vi "Seq Test Editor.vi"(6 "User Name":string="zhangxf", 8 "Sys Error":errorcluster, 9 "Part Type":string="ALL Type", 10 "Station":string="FA03", 11 "Base Path":path=path "C:/Labview Code") -> (0 "Sys Error Out":errorcluster)   [LabVIEW 2018]
uses:
  type defs/Sequence Info.ctl
  type defs/Sequence Status.ctl
  type defs/Sequence paths.ctl
  type defs/config paths for seq def.ctl
  <vilib>/Utility/file.llb/Write To Spreadsheet File (string).vi
panel:
  in  "Save":bool
  out "Sequence Name":string="F15 Audit 1 Sequence"
  in  "Exit":bool
  in  "Sequence":i32(listbox)=7
  in  "Steps":i32(listbox)
  in  "Edit Step":bool
  in  "Up":bool
  in  "Down":bool
  in  "Copy Step":bool
  in  "Delete":bool
  in  "Insert Step":bool
  # "[Page Up]"
  # "[Page Dn]"
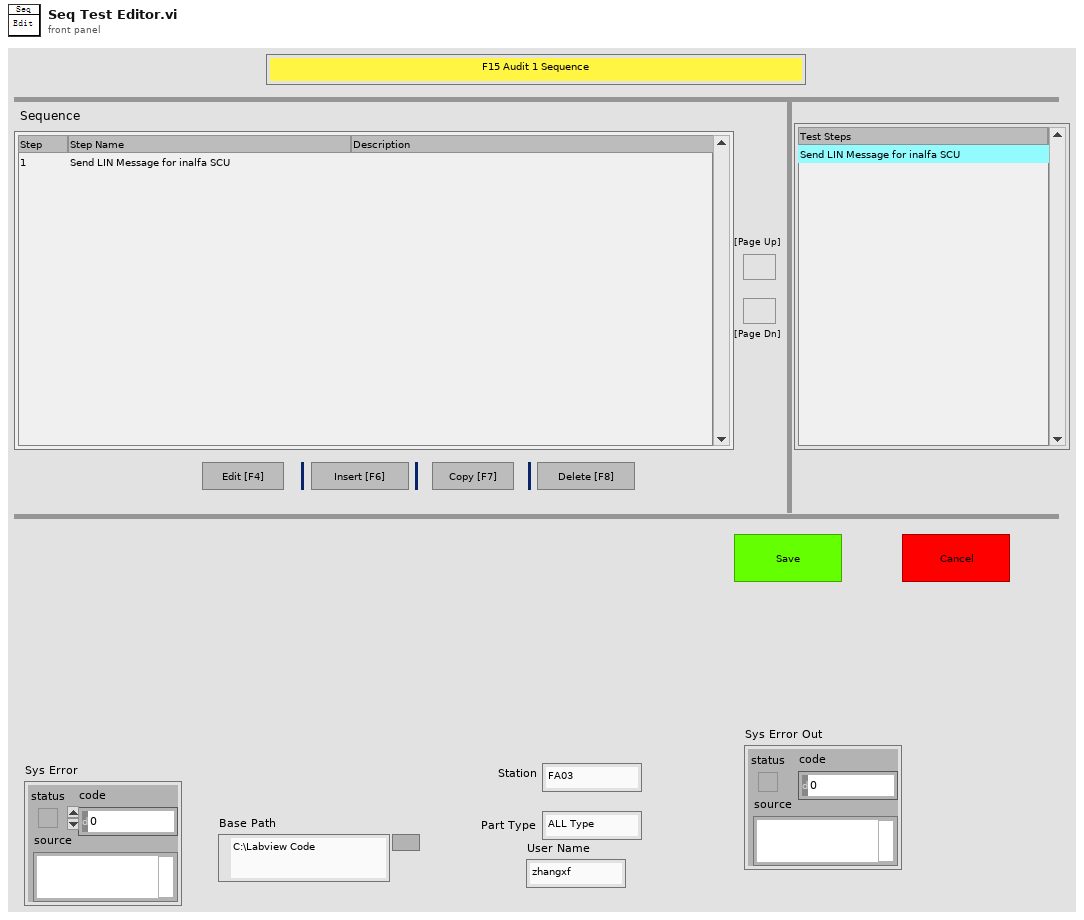
[diagram p1: front panel]
types:
  T1 = typedef "Sequence paths.ctl" = cluster{"Sequence Path":path, "Sequence Histroy Path":path, "Current Sequence Path":path, "Sequence Config Path":path, "Sequence VI's Path":path}
  T2 = typedef "Sequence Status.ctl" = enum16{"No Change", "Edited", "New Step", "Deleted", "Moved Up", "Moved Down", "Copied"}
  T3 = typedef "Sequence Info.ctl" = cluster{"Name":string, "Description":string, "data string":string}
  T4 = cluster{"Paths of Sequence":T1, "Type":string, "Sequence Name:":i32, "Sequence":refnum<vi>, "Steps":refnum<vi>, "Sequence Info":T3[], "Sequence Scroll":u32, "Basic Steps":string[], "Sequences":string[], "Sequence Text":string, "Station":string, "New Step?":bool, "Part Type":string, "User Name":string, "Sequence History":string[][], "Sequence Status":T2, "Sequence History Index":i32, "Step History Data":string[], "VI Names":string[], "Sys Error":errorcluster, "Current Sequence":string[][], "Base Path":path, "Description":string[]}
  T5 = typedef "config paths for seq def.ctl" = cluster{"Part Type":string, "base path":path, "Seq VI's path":path}
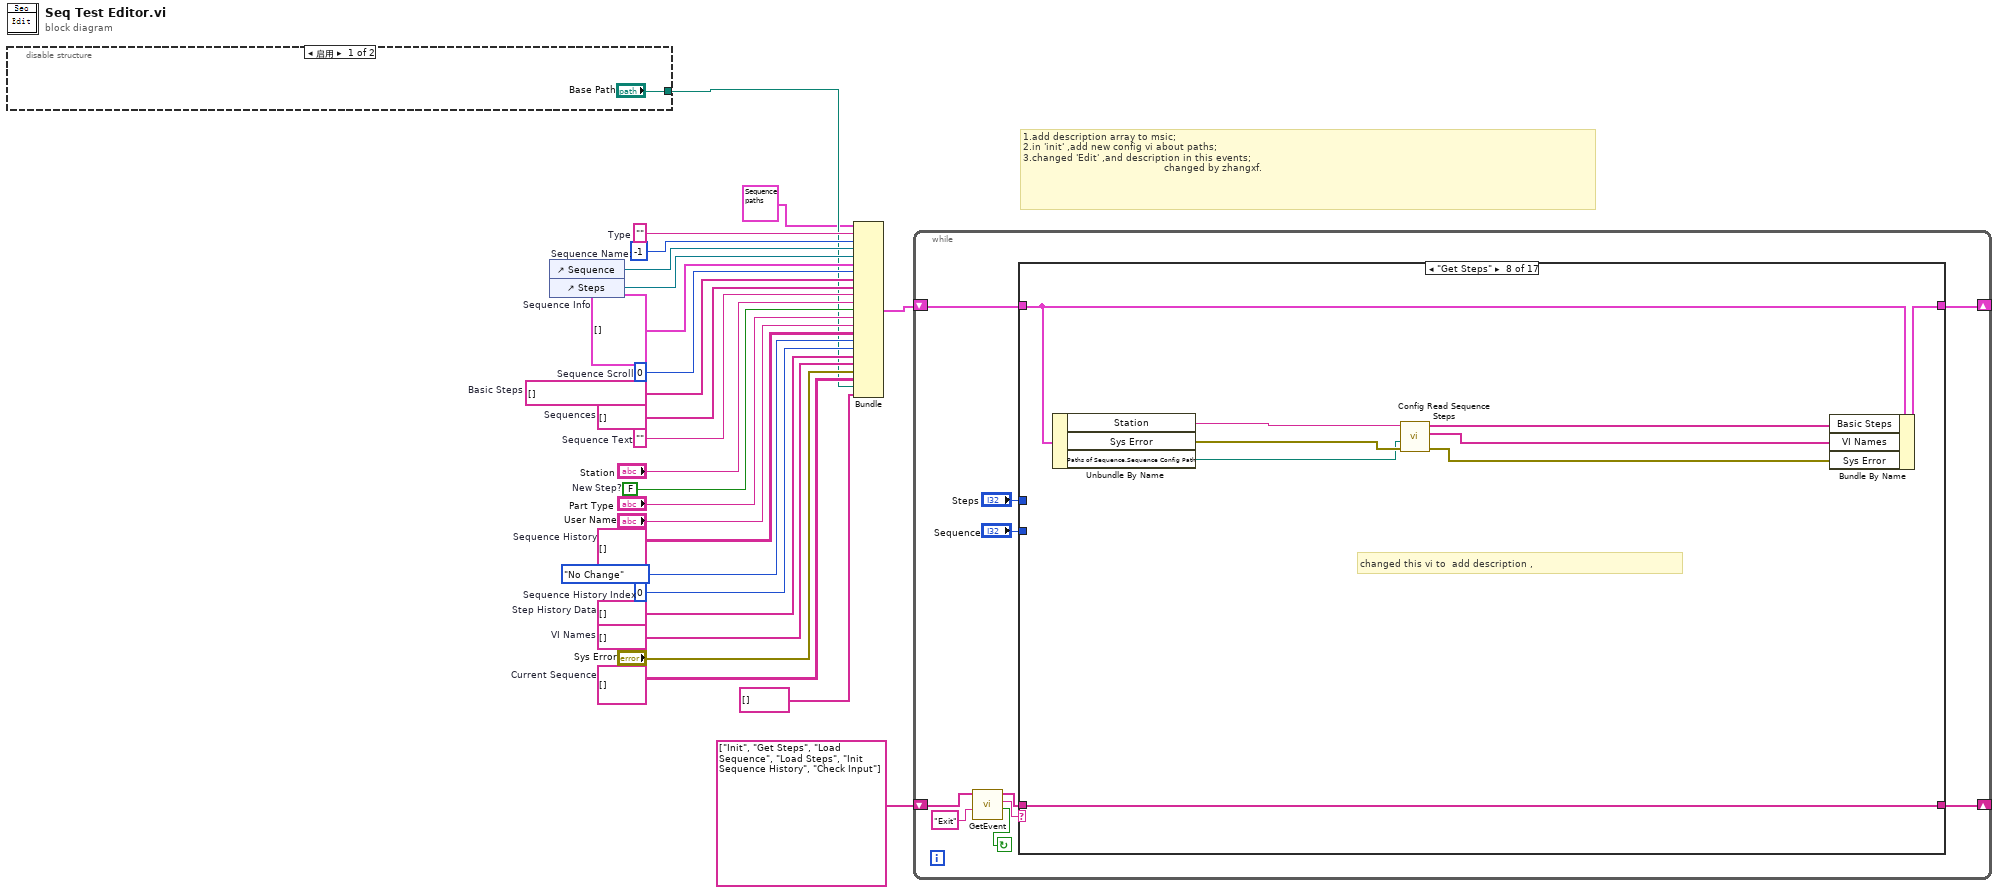
[diagram p0: block diagram]
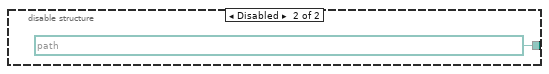
[diagram p2: hidden frame]
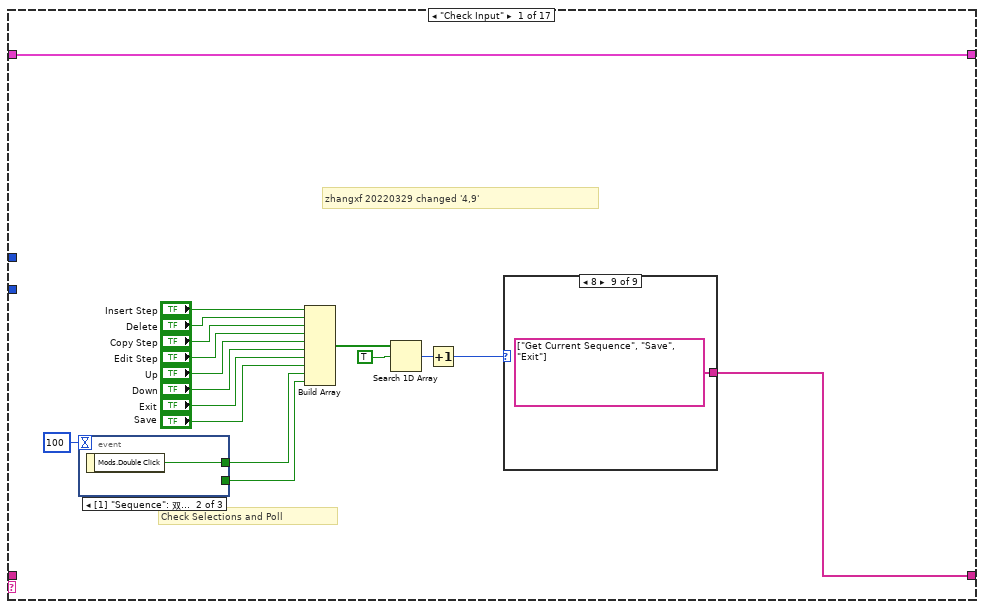
[diagram p3: hidden frame]
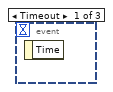
[diagram p4: hidden frame]
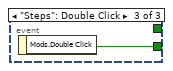
[diagram p5: hidden frame]
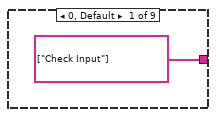
[diagram p6: hidden frame]
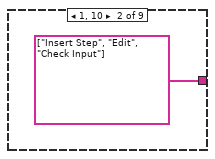
[diagram p7: hidden frame]
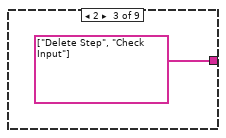
[diagram p8: hidden frame]
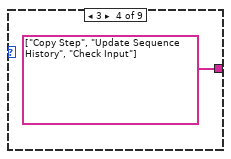
[diagram p9: hidden frame]
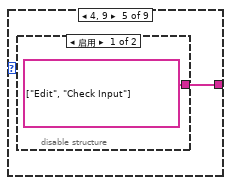
[diagram p10: hidden frame]
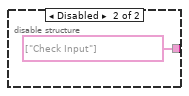
[diagram p11: hidden frame]
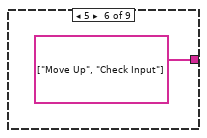
[diagram p12: hidden frame]
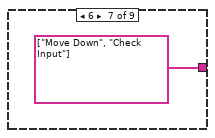
[diagram p13: hidden frame]
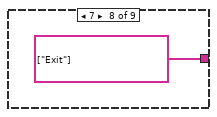
[diagram p14: hidden frame]
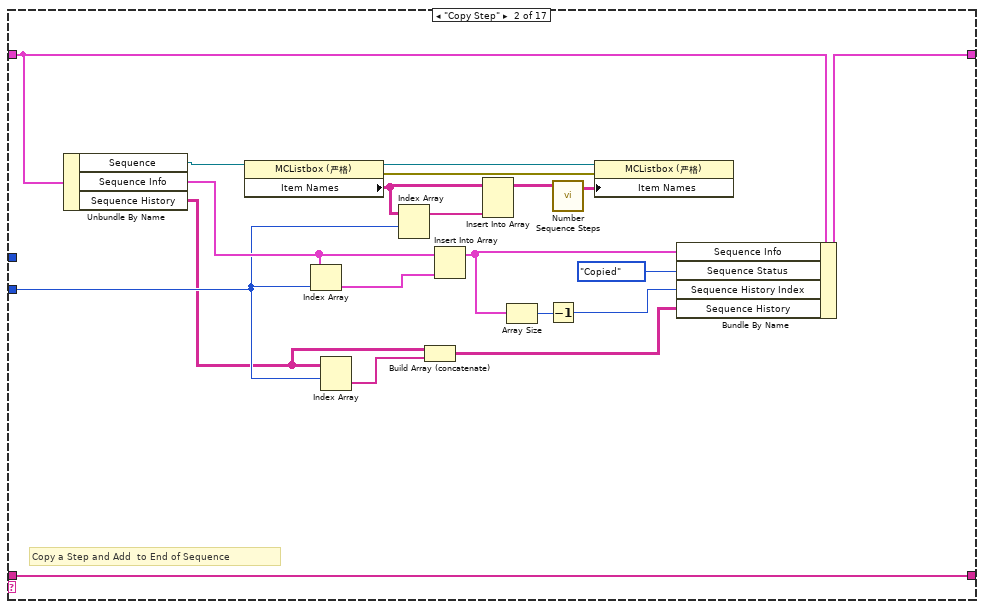
[diagram p15: hidden frame]
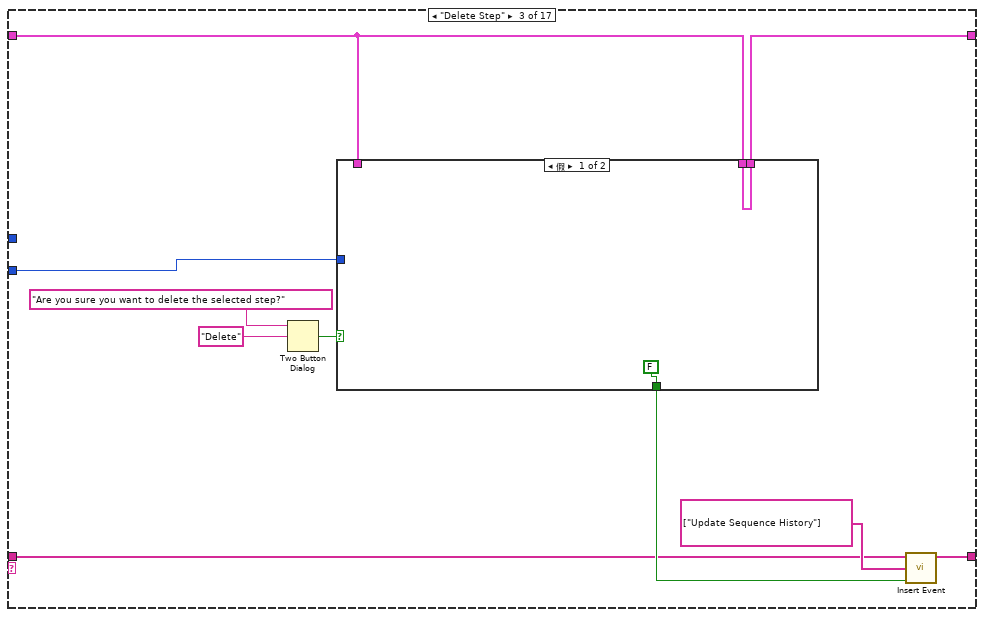
[diagram p16: hidden frame]
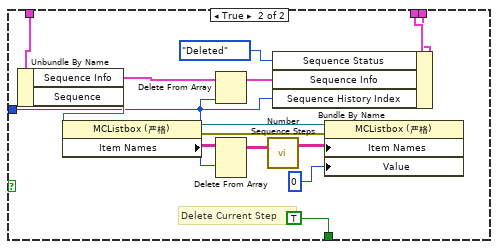
[diagram p17: hidden frame]
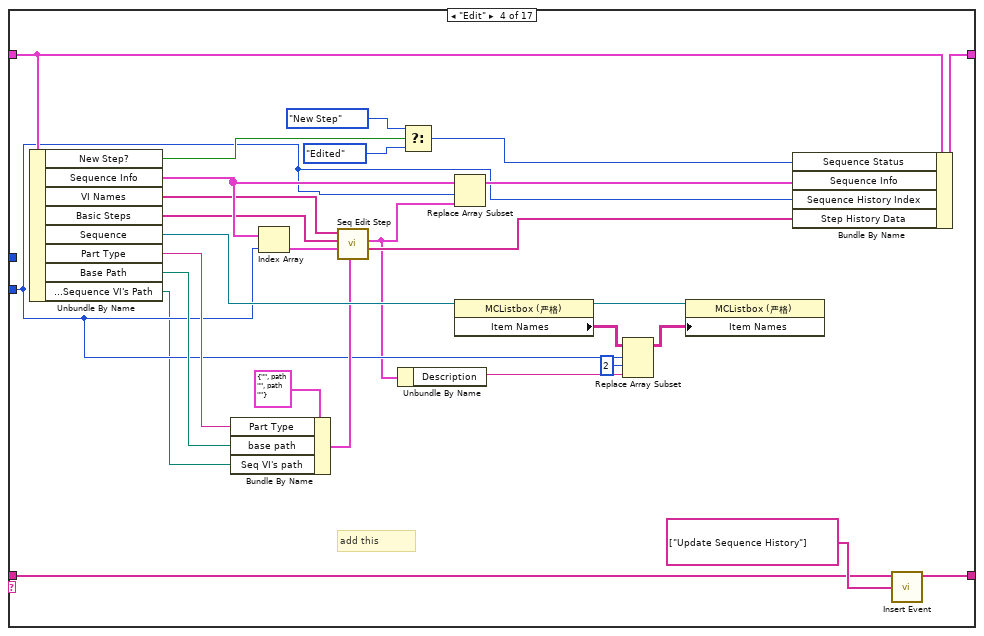
[diagram p18: hidden frame]
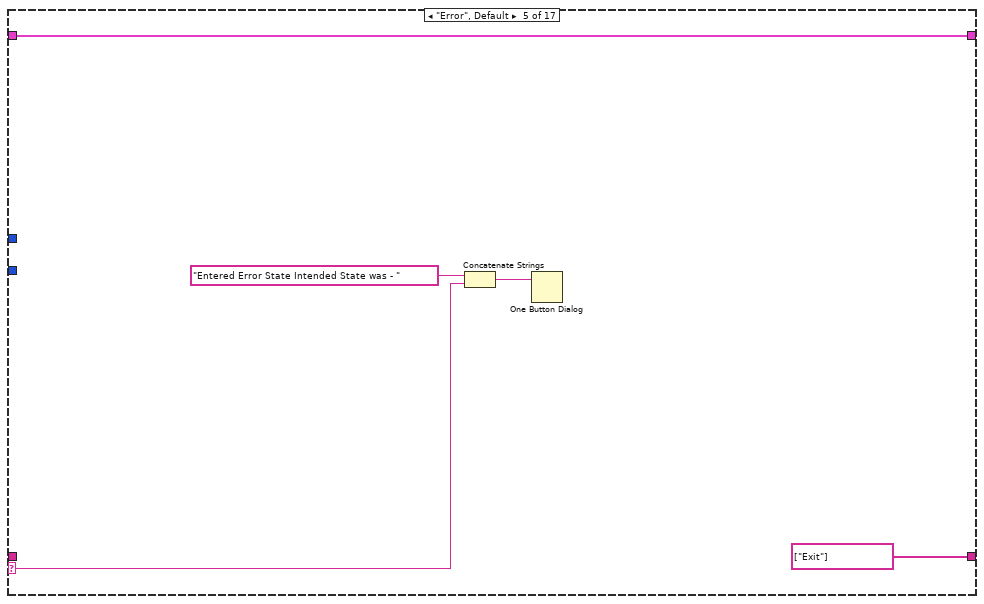
[diagram p19: hidden frame]
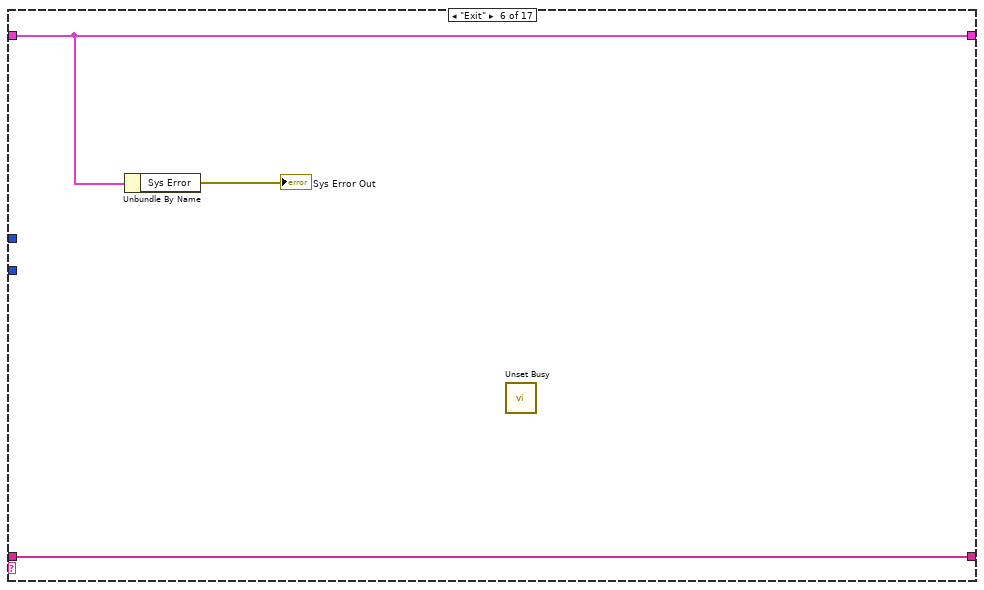
[diagram p20: hidden frame]
diagram:
  w4 = string[][] []  # Current Sequence
  w6 = string[] []  # VI Names
  w7 = string[] []  # Step History Data
  w8 = 0  # Sequence History Index
  w15 = FALSE  # New Step?
  w10 = string[][] []  # Sequence History
  w13 = T3[] []  # Sequence Info
  w17 = string[] []  # Sequences
  w19 = ""  # Sequence Text
  w20 = -1  # Sequence Name:
  w16 = string[] []  # Basic Steps
  w22 = u32 0  # Sequence Scroll
  w18 = ""  # Type
  # "1.add description array to msic;\n2.in 'init' ,add new config vi about paths;\n3.changed 'Edit' ,and description in this events;\n                                               changed by zhangxf."
  n1 = disable-structure shown="启用" {
    disable-tunnel: ["Base Path" path "D:/工作盘/116所/RD246/NI/RD246_MES/Mobitech_MES/System/Part Configuration" ("Base Path")] -> w3
    frame Enabled {
    }
    frame Disabled {
    }
  }
  n2 = control-ref of="Sequence"() -> (w23:refnum<vi>)
  n3 = control-ref of="Steps"() -> (w21:refnum<vi>)
  n4 = Bundle("Paths of Sequence"=T1 {"Sequence Path"=path "", "Sequence Histroy Path"=path "", "Current Sequence Path"=path "", "Sequence Config Path"=path "", "Sequence VI's Path"=path ""}, "Type"=w18, "Sequence Name:"=w20, "Sequence"=w23, "Steps"=w21, "Sequence Info"=w13, "Sequence Scroll"=w22, "Basic Steps"=w16, "Sequences"=w17, "Sequence Text"=w19, "Station"="Station", "New Step?"=w15, "Part Type"="Part Type", "User Name"="User Name", "Sequence History"=w10, "Sequence Status"=Sequence_Status."No Change", "Sequence History Index"=w8, "Step History Data"=w7, "VI Names"=w6, "Sys Error"="Sys Error", "Current Sequence"=w4, "Base Path"=w3, "Description"=string[] []) -> (w24:T4)  [unwired: 1 in]
  n5 = while {
    shift-right: [w37] -> _
    shift-left: string[] ["Init", "Get Steps", "Load Sequence", "Load Steps", "Init Sequence History", "Check Input"] -> [w32]
    shift-right: [w35] -> _
    shift-left: w24 -> [w36]
    stop <- w30 continue-if-true
    n6 = call "GetEvent.vi"("标志事件"="Exit" ("Exit Event"), "事件组"=w32) -> ("？"=w30:bool, "下一事件"=w28:string, "下一事件组"=w29:string[])  [unwired: 3 in, 2 out]
    n7 = case shown="\"Get Steps\"" w28 {
      selector: w28 -> [_ _ _ _ w144 _ _ _ _ _ _ _ _ _ _ _ _]
      tunnel: w29 -> [_ w80 w88 w129 _ w150 w162 w183 w193 w208 w224 w256 w264 w266 w302 w335 w350]
      tunnel: [w47 w80 w89 w130 string[] ["Exit"] ("event queue out") w150 w162 w183 w193 w208 w224 w256 w264 w267 w301 w335 w350] -> w37
      tunnel: w36 -> [w40 w82 w94 w142 w147 w149 w158 w182 w185 w198 w234 w254 w259 w277 w304 w340 w347]
      tunnel: [w40 w81 w93 w141 w147 w149 w157 w181 w186 w197 w233 w258 w259 w279 w306 w340 w349] -> w35
      tunnel: "Steps" -> [_ _ _ _ _ _ _ _ _ _ w220 _ _ _ _ _ _]
      tunnel: "Sequence" -> [_ w72 w92 w119 _ _ _ _ _ _ w223 _ _ w271 w305 _ _]
      frame "Check Input" {
        # "zhangxf 20220329 changed '4,9'"
        # "Check Selections and Poll"
        n8 = event shown="[1] \"Sequence\": 双击" {
          selector: _ -> [_ _ _]
          dyn-events: _ -> [_ _ _]
          timeout: 100 -> [_ _ _]
          tunnel: [_ w55 _] -> w44
          tunnel: [_ _ w56] -> w43
          event Timeout {
            n9 = event-data() -> ()  [unwired: 1 in, 1 out]
          }
          event "Sequence": Double Click {
            n10 = event-data() -> ("Mods.Double Click"=w55:bool)  [unwired: 1 in]
          }
          event "Steps": Double Click {
            n11 = event-data() -> ("Mods.Double Click"=w56:bool)  [unwired: 1 in]
          }
        }
        n12 = Build Array("Insert Step", "Delete", "Copy Step", "Edit Step", "Up", "Down", "Exit", "Save", w44, w43) -> (w50:bool[])
        n13 = Search 1D Array(1D array=w50, element=TRUE) -> (index of element=w49:i32)  [unwired: 1 in]
        n14 = Increment(x=w49) -> (x+1=w38:i32)
        n15 = case shown="8" w38 {
          tunnel: [string[] ["Check Input"] string[] ["Insert Step", "Edit", "Check Input"] string[] ["Delete Step", "Check Input"] string[] ["Copy Step", "Update Sequence History", "Check Input"] w61 string[] ["Move Up", "Check Input"] string[] ["Move Down", "Check Input"] string[] ["Exit"] string[] ["Get Current Sequence", "Save", "Exit"]] -> w47
          frame 0, Default {
          }
          frame 1, 10 {
          }
          frame 2 {
          }
          frame 3 {
          }
          frame 4, 9 {
            n16 = disable-structure shown="启用" {
              disable-tunnel: [string[] ["Edit", "Check Input"] string[] ["Check Input"]] -> w61
              frame Enabled {
              }
              frame Disabled {
              }
            }
          }
          frame 5 {
          }
          frame 6 {
          }
          frame 7 {
          }
          frame 8 {
          }
        }
      }
      frame "Copy Step" {
        # "Copy a Step and Add  to End of Sequence"
        n17 = Unbundle By Name(w82) -> ("Sequence"=w87:refnum<vi>, "Sequence Info"=w77:T3[], "Sequence History"=w71:string[][])
        n18 = property class="MCListbox (严格)"(reference=w87) -> (reference out=w84:refnum<vi>, error out=w83:errorcluster, "Item Names"=w79:string[][])  [unwired: 1 in]
        n19 = Index Array(array=w77, index=w72) -> (element=w76:T3)
        n20 = Index Array(array=w71, index (row)=w72) -> (element=w70:string[])  [unwired: 1 in]
        n21 = Index Array(array=w79, index (row)=w72) -> (element=w78:string[])  [unwired: 1 in]
        n22 = Build Array (concatenate)(w71, w70) -> (w69:string[][])
        n23 = Insert Into Array(array=w77, new element=w76) -> (w68:T3[])  [unwired: 1 in]
        n24 = Insert Into Array(array=w79, new element=w78) -> (w86:string[][])  [unwired: 2 in]
        n25 = Array Size(array=w68) -> (size(s)=w74:i32)
        n26 = Decrement(x=w74) -> (x-1=w73:i32)
        n27 = call "Number Sequence Steps.vi"("Sequence Names"=w86) -> ("ItemNames Out"=w85:string[][])  [unwired: 1 out]
        n28 = property class="MCListbox (严格)"(reference=w84, error in=w83, "Item Names"=w85) -> ()  [unwired: 2 out]
        n29 = Bundle By Name(cluster=w82, "Sequence Info"=w68, "Sequence Status"=Sequence_Status."Copied", "Sequence History Index"=w73, "Sequence History"=w69) -> (w81:T4)
      }
      frame "Delete Step" {
        n30 = Two Button Dialog(message="Are you sure you want to delete the selected step?", 2:"Delete" ("T button name (\"OK\")")) -> (T button?=w95:bool)  [unwired: 1 in]
        n31 = case shown="假" w95 {
          tunnel: w94 -> [_ w114]
          tunnel: w94 -> [w99 w112]
          tunnel: [w99 w111] -> w93
          tunnel: w92 -> [_ w101]
          tunnel: [FALSE TRUE] -> w90
          frame False {
          }
          frame True {
            # "Delete Current Step"
            n32 = Unbundle By Name(w114) -> ("Sequence Info"=w110:T3[], "Sequence"=w113:refnum<vi>)
            n33 = property class="MCListbox (严格)"(reference=w113) -> (reference out=w107:refnum<vi>, error out=w106:errorcluster, "Item Names"=w108:string[][])  [unwired: 1 in]
            n34 = Delete From Array(array=w110, index=w101) -> (array with subset deleted=w109:T3[])  [unwired: 1 in, 1 out]
            n35 = Delete From Array(array=w108, index (row)=w101) -> (array with subset deleted=w105:string[][])  [unwired: 2 in, 1 out]
            n36 = call "Number Sequence Steps.vi"("Sequence Names"=w105) -> ("ItemNames Out"=w104:string[][])  [unwired: 1 out]
            n37 = Bundle By Name(cluster=w112, "Sequence Status"=Sequence_Status."Deleted", "Sequence Info"=w109, "Sequence History Index"=w101) -> (w111:T4)
            n38 = property class="MCListbox (严格)"(reference=w107, error in=w106, "Item Names"=w104, "Value"=0) -> ()  [unwired: 2 out]
          }
        }
        n39 = call "Insert Event.vi"("Event queue in"=w88, "Insert all? (T)"=w90, "Events to Insert"=string[] ["Update Sequence History"]) -> ("Event queue out"=w89:string[])  [unwired: 7 in]
      }
      frame "Edit" {
        # "add this"
        n40 = Unbundle By Name(w142) -> ("New Step?"=w136:bool, "Sequence Info"=w139:T3[], "VI Names"=w128:string[], "Basic Steps"=w126:string[], "Sequence"=w127:refnum<vi>, "Part Type"=w124:string, "Base Path"=w123:path, "Paths of Sequence.Sequence VI's Path"=w115:path)
        n41 = Bundle By Name(cluster=T5 {"Part Type"="", "base path"=path "", "Seq VI's path"=path ""} ("config paths"), "Part Type"=w124, "base path"=w123, "Seq VI's path"=w115) -> (w122:T5)
        n42 = Index Array(array=w139, index=w119) -> (element=w137:T3)
        n43 = call "Seq Edit Step.vi"("config paths"=w122, "Segment Info In"=w137, "Basic Steps"=w126, "VI Names"=w128) -> ("Step Hisitory"=w132:string[], "Segment Info Out"=w118:T3)  [unwired: 4 in, 2 out]
        n44 = Unbundle By Name(w118) -> ("Description"=w117:string)
        n45 = Select(t=Sequence_Status."New Step" ("Sequence Status"), s=w136, f=Sequence_Status."Edited" ("Sequence Status")) -> (s? t:f=w133:T2)
        n46 = Replace Array Subset(array=w139, new element=w118, index=w119) -> (w140:T3[])
        n47 = property class="MCListbox (严格)"(reference=w127) -> (reference out=w138:refnum<vi>, "Item Names"=w121:string[][])  [unwired: 1 in, 1 out]
        n48 = Replace Array Subset(array=w121, new element=w117, index (row)=w119, index (col)=2 ("禁用的索引 (列)")) -> (w120:string[][])
        n49 = property class="MCListbox (严格)"(reference=w138, "Item Names"=w120) -> ()  [unwired: 1 in, 2 out]
        n50 = Bundle By Name(cluster=w142, "Sequence Status"=w133, "Sequence Info"=w140, "Sequence History Index"=w119, "Step History Data"=w132) -> (w141:T4)
        n51 = call "Insert Event.vi"("Event queue in"=w129, "Events to Insert"=string[] ["Update Sequence History"]) -> ("Event queue out"=w130:string[])  [unwired: 8 in]
      }
      frame "Error", Default {
        n52 = Concatenate Strings("Entered Error State Intended State was - " ("string"), w144) -> (w143:string)
        n53 = One Button Dialog(message=w143) -> ()  [unwired: 1 in, 1 out]
      }
      frame "Exit" {
        n54 = Unbundle By Name(w149) -> ("Sys Error"=→"Sys Error Out":errorcluster)
        n55 = call <vilib>:"Unset Busy.vi"() -> ()  [unwired: 11 in, 1 out]
      }
      frame "Get Current Sequence" {
        n56 = Unbundle By Name(w158) -> ("VI Names"=w159:string[], "Basic Steps"=w160:string[], "Sequence Info"=w161:T3[], "Part Type"=w154:string, "Base Path"=w153:path, "Paths of Sequence.Sequence VI's Path"=w151:path)
        n57 = Bundle By Name(cluster=T5 {"Part Type"="", "base path"=path "", "Seq VI's path"=path ""} ("config paths"), "Part Type"=w154, "base path"=w153, "Seq VI's path"=w151) -> (w152:T5)
        n58 = for {
          tunnel: w161 -> [w174] mode=indexing
          tunnel: w160 -> [w173]
          tunnel: w159 -> [w172]
          tunnel: [w167] -> w156 mode=indexing
          tunnel: w152 -> [w163]
          n59 = call "Seq Get Current Sequence.vi"("config paths"=w163, "Segment Info In"=w174, "Basic Steps"=w173, "VI Names"=w172) -> ("Step Hisitory"=w171:string[])  [unwired: 6 in, 1 out]
          n60 = Index Array(array=w171, index #1=0 ("index"), index #2=3 ("index"), index #3=1 ("index")) -> (element #1=w170:string, element #2=w169:string, element #3=w168:string)
          n61 = Build Array(w170, w169, w168) -> (w167:string[])
        }
        n62 = call <vilib>:"Set Busy.vi"() -> ()  [unwired: 10 in, 2 out]
        n63 = Bundle By Name(cluster=w158, "Current Sequence"=w156) -> (w157:T4)
      }
      frame "Get Steps" {
        # "changed this vi to  add description ,"
        n64 = Unbundle By Name(w182) -> ("Station"=w180:string, "Sys Error"=w177:errorcluster, "Paths of Sequence.Sequence Config Path"=w175:path)
        n65 = call "Config Read Sequence Steps.vi"("Error In"=w177, "Base Path"=w175, "Station Name"=w180) -> ("Error Out"=w176:errorcluster, "VI Names"=w178:string[], "Sequence Steps"=w179:string[])  [unwired: 6 in]
        n66 = Bundle By Name(cluster=w182, "Basic Steps"=w179, "VI Names"=w178, "Sys Error"=w176) -> (w181:T4)
      }
      frame "Init" {
        w190 = string[][] [] ("Item Names")
        w189 = u32 9567230
        w188 = 0 ("Value")
        # "add this vi to config paths"
        n67 = Unbundle By Name(w185) -> ("Sequence"=w192:refnum<vi>, "Steps"=w191:refnum<vi>)
        n68 = call "Creat file for Seq path.vi"("ini in"=w185) -> ("Paths of Sequence"=w184:T1)  [unwired: 10 in]
        n69 = property class="MCListbox (严格)"(reference=w192, "Item Names"=w190, "Value"=w188, "Selection Color"=w189) -> ()  [unwired: 1 in, 2 out]
        n70 = property class="MCListbox (严格)"(reference=w191, "Item Names"=w190, "Value"=w188, "Selection Color"=w189, "Disabled Items"=i32[] []) -> ()  [unwired: 1 in, 2 out]
        n71 = Bundle By Name(cluster=w185, "Paths of Sequence"=w184) -> (w186:T4)
      }
      frame "Init Sequence History" {
        n72 = Unbundle By Name(w198) -> ("User Name"=w202:string, "Part Type"=w204:string, "Station"=w206:string, "Sequence Info"=w207:T3[], "Sequence Status"=w195:T2)
        n73 = Get Date/Time String() -> (date string=w200:string, time string=w201:string)  [unwired: 3 in]
        n74 = Format Into String(w204) -> (resulting string=w203:string)  [unwired: 3 in, 1 out]
        n75 = Format Into String(w206) -> (resulting string=w205:string)  [unwired: 3 in, 1 out]
        n76 = Format Into String(w195) -> (resulting string=w199:string)  [unwired: 3 in, 1 out]
        n77 = for {
          tunnel: w207 -> [w218] mode=indexing
          tunnel: w205 -> [w213]
          tunnel: w203 -> [w214]
          tunnel: w202 -> [w215]
          tunnel: w201 -> [w216]
          tunnel: w200 -> [w217]
          tunnel: [w211] -> w196 mode=indexing
          tunnel: w199 -> [w210]
          tunnel: "NA" -> [w209]
          n78 = Unbundle By Name(w218) -> ("Name"=w212:string)
          n79 = Build Array(w215, w217, w216, w214, w213, w212, w210, w209, w209) -> (w211:string[])
        }
        n80 = Bundle By Name(cluster=w198, "Sequence History"=w196) -> (w197:T4)
      }
      frame "Insert Step" {
        # "zhangxf 20220328 changed: This change causes the new \nstep to be inserted downward"
        # "zhangxf 20220328 changed: add description in items"
        n81 = Unbundle By Name(w234) -> ("Sequence"=w242:refnum<vi>, "Steps"=w245:refnum<vi>, "Sequence Info"=w229:T3[], "Description"=w221:string[])
        n82 = property class="MCListbox (严格)"(reference=w245) -> (error out=w241:errorcluster, "Item Names"=w244:string[][])  [unwired: 1 in, 1 out]
        n83 = Index Array(array=w221, index=w220) -> (element=w219:string)
        n84 = case shown="..-1" w223 {
          selector: w223 -> [w247 _]
          tunnel: [w246 0 ("Sequence")] -> w222
          frame 0.. {
            n85 = Increment(x=w247) -> (x+1=w246:i32)
          }
          frame ..-1 {
          }
        }
        n86 = Index Array(array=w244, index (row)=w220, index (col)=0 ("disabled index (col)")) -> (element=w228:string)
        n87 = property class="MCListbox (严格)"(reference=w242, error in=w241) -> (reference out=w236:refnum<vi>, error out=w235:errorcluster, "Item Names"=w239:string[][])
        n88 = Bundle By Name(cluster=T3 {"Name"="", "Description"="", "data string"=""} ("Segment Data"), "Name"=w228, "Description"=w219) -> (w231:T3)
        n89 = Build Array("1" ("element"), w228, "") -> (w238:string[])
        n90 = Insert Into Array(array=w239, index (row)=w222, new element=w238) -> (w240:string[][])  [unwired: 1 in]
        n91 = Insert Into Array(array=w229, index=w222, new element=w231) -> (w230:T3[])
        n92 = call "Number Sequence Steps.vi"("Sequence Names"=w240) -> ("ItemNames Out"=w237:string[][])  [unwired: 1 out]
        n93 = property class="MCListbox (严格)"(reference=w236, error in=w235, "Item Names"=w237, "Value"=w222) -> ()  [unwired: 2 out]
        n94 = Bundle By Name(cluster=w234, "Sequence Info"=w230, "New Step?"=TRUE) -> (w233:T4)
      }
      frame "Load Sequence" {
        # "Load Sequence"
        n95 = Unbundle By Name(w254) -> ("Sequence"=w257:refnum<vi>, "Part Type"=w250:string, "Station"=w251:string, "Paths of Sequence.Sequence Path"=w249:path)
        n96 = call "Config Load Sequence.vi"("Base Path"=w249, "Station"=w251, "Part Type"=w250) -> ("Sequence Name"=→"Sequence Name":string, "Item Names"=w255:string[][], "Seqence Info"=w253:T3[])  [unwired: 5 in, 1 out]
        n97 = property class="MCListbox (严格)"(reference=w257, "Item Names"=w255) -> ()  [unwired: 1 in, 2 out]
        n98 = Bundle By Name(cluster=w254, "Sequence Info"=w253) -> (w258:T4)
      }
      frame "Load Steps" {
        n99 = Unbundle By Name(w259) -> ("Steps"=w263:refnum<vi>, "Basic Steps"=w262:string[])
        n100 = Build Array(w262) -> (w261:string[][])
        n101 = Transpose 2D Array(2D array=w261) -> (transposed array=w260:string[][])
        n102 = property class="MCListbox (严格)"(reference=w263, "Item Names"=w260) -> ()  [unwired: 1 in, 2 out]
      }
      frame "Move Down" {
        # "Move the step Down one in the sequence"
        n103 = Unbundle By Name(w277) -> ("Sequence Info"=w276:T3[], "Sequence"=w275:refnum<vi>)
        n104 = property class="MCListbox (严格)"(reference=w275) -> (reference out=w280:refnum<vi>, error out=w278:errorcluster, "Item Names"=w274:string[][])  [unwired: 1 in]
        n105 = Array Size(array=w274) -> (size(s)=w273:i32[])
        n106 = Index Array(array=w273) -> (element=w272:i32)  [unwired: 1 in]
        n107 = Decrement(x=w272) -> (x-1=w269:i32)
        n108 = Greater?(x=w269, y=w271) -> (0:w270:bool)
        n109 = case shown="真" w270 {
          tunnel: w280 -> [_ w299]
          tunnel: [w282 w298] -> w279
          tunnel: w278 -> [_ w297]
          tunnel: w277 -> [w282 w296]
          tunnel: w276 -> [_ w295]
          tunnel: w274 -> [_ w291]
          tunnel: w271 -> [_ w284]
          tunnel: [FALSE TRUE] -> w265
          frame False {
            # "At Bottom"
          }
          frame True {
            # "Move Down"
            n110 = Delete From Array(array=w295, index=w284) -> (deleted portion=w293:T3, array with subset deleted=w294:T3[])  [unwired: 1 in]
            n111 = Delete From Array(array=w291, index (row)=w284) -> (deleted portion=w289:string[], array with subset deleted=w290:string[][])  [unwired: 2 in]
            n112 = Increment(x=w284) -> (x+1=w288:i32)
            n113 = Insert Into Array(array=w294, index=w288, new element=w293) -> (w292:T3[])
            n114 = Insert Into Array(array=w290, index (row)=w288, new element=w289) -> (w287:string[][])  [unwired: 1 in]
            n115 = Bundle By Name(cluster=w296, "Sequence Status"=Sequence_Status."Moved Down", "Sequence Info"=w292, "Sequence History Index"=w284) -> (w298:T4)
            n116 = call "Number Sequence Steps.vi"("Sequence Names"=w287) -> ("ItemNames Out"=w286:string[][])  [unwired: 1 out]
            n117 = property class="MCListbox (严格)"(reference=w299, error in=w297, "Item Names"=w286, "Value"=w288) -> ()  [unwired: 2 out]
          }
        }
        n118 = call "Insert Event.vi"("Event queue in"=w266, "Insert all? (T)"=w265, "Events to Insert"=string[] ["Update Sequence History"]) -> ("Event queue out"=w267:string[])  [unwired: 7 in]
      }
      frame "Move Up" {
        # "Move the Step Up one in the Sequence"
        n119 = case shown="1, 默认" w305 {
          selector: w305 -> [_ w310]
          tunnel: [w308 w326] -> w306
          tunnel: w304 -> [w308 w316]
          tunnel: w304 -> [_ w315]
          tunnel: [FALSE TRUE] -> w300
          frame 0 {
            # "Do Not Move Up If at Top"
          }
          frame 1, Default {
            # "Move Up"
            n120 = Unbundle By Name(w315) -> ("Sequence Info"=w324:T3[], "Sequence"=w322:refnum<vi>)
            n121 = property class="MCListbox (严格)"(reference=w322) -> (reference out=w327:refnum<vi>, error out=w325:errorcluster, "Item Names"=w319:string[][])  [unwired: 1 in]
            n122 = Delete From Array(array=w324, index=w310) -> (deleted portion=w321:T3, array with subset deleted=w323:T3[])  [unwired: 1 in]
            n123 = Delete From Array(array=w319, index (row)=w310) -> (deleted portion=w317:string[], array with subset deleted=w318:string[][])  [unwired: 2 in]
            n124 = Decrement(x=w310) -> (x-1=w311:i32)
            n125 = Insert Into Array(array=w323, index=w311, new element=w321) -> (w320:T3[])
            n126 = Insert Into Array(array=w318, index (row)=w311, new element=w317) -> (w314:string[][])  [unwired: 1 in]
            n127 = Bundle By Name(cluster=w316, "Sequence Status"=Sequence_Status."Moved Up", "Sequence Info"=w320, "Sequence History Index"=w310) -> (w326:T4)
            n128 = call "Number Sequence Steps.vi"("Sequence Names"=w314) -> ("ItemNames Out"=w313:string[][])  [unwired: 1 out]
            n129 = property class="MCListbox (严格)"(reference=w327, error in=w325, "Item Names"=w313, "Value"=w311) -> ()  [unwired: 2 out]
          }
        }
        n130 = call "Insert Event.vi"("Event queue in"=w302, "Insert all? (T)"=w300, "Events to Insert"=string[] ["Update Sequence History"]) -> ("Event queue out"=w301:string[])  [unwired: 7 in]
      }
      frame "Save" {
        n131 = Unbundle By Name(w340) -> ("Paths of Sequence.Sequence Histroy Path"=w330:path, "Paths of Sequence.Sequence Path"=w328:path, "Sequence Info"=w332:T3[], "Sequence History"=w331:string[][], "Current Sequence"=w333:string[][], "Paths of Sequence.Current Sequence Path"=w329:path)  [unwired: 2 out]
        n132 = Build Array("\n") -> (w336:string[])
        n133 = Flatten To String(anything=w332) -> (data string=w339:string)  [unwired: 3 in, 2 out]
        n134 = Build Array (concatenate)(w331, w336) -> (w334:string[][])
        n135 = call-poly <vilib>:"Write To Spreadsheet File.vi"("2D data"=w333, "file path (dialog if empty)"=w329) -> ()  [unwired: 6 in, 1 out]
        n136 = call "Write Characters To File with Advisory Dialog Option.vi"("character string"=w339, "file path (dialog if empty)"=w328) -> ()  [unwired: 8 in, 2 out]
        n137 = call-poly <vilib>:"Write To Spreadsheet File.vi"("append to file? (new file:F)"=TRUE, "2D data"=w334, "file path (dialog if empty)"=w330) -> ()  [unwired: 5 in, 1 out]
      }
      frame "Update Sequence History" {
        n138 = Unbundle By Name(w347) -> ("Sequence History"=w346:string[][], "Sequence Status"=w342:T2, "Sequence History Index"=w345:i32, "Step History Data"=w344:string[])
        n139 = Format Into String(w342) -> (resulting string=w341:string)  [unwired: 3 in, 1 out]
        n140 = case shown="\"Moved Up\"" w342 {
          tunnel: w346 -> [w351 w355 w373 w389 w398 w408 w416]
          tunnel: w345 -> [_ w354 w372 w388 w397 w407 w415]
          tunnel: w344 -> [_ w363 w380 _ _ _ _]
          tunnel: [w351 w353 w371 w387 w396 w401 w409] -> w343
          tunnel: w341 -> [_ w352 w366 w385 w394 w404 w412]
          frame "No Change", Default {
          }
          frame "Edited" {
            n141 = Index Array(array=w355, index (row)=w354) -> (element=w365:string[])  [unwired: 1 in]
            n142 = Index Array(array=w363) -> (element #2=w358:string, element #3=w357:string)  [unwired: 3 in, 1 out]
            n143 = Replace Array Subset(array=w365, new element=w352, index=6) -> (w362:string[])
            n144 = Replace Array Subset(array=w362, new element=w358, index=7) -> (w361:string[])
            n145 = Replace Array Subset(array=w361, new element=w357, index=8) -> (w356:string[])
            n146 = Replace Array Subset(array=w355, new element=w356, index (row)=w354) -> (w353:string[][])  [unwired: 1 in]
          }
          frame "New Step" {
            n147 = Index Array(array=w373, index (row)=w372) -> (element=w382:string[])  [unwired: 1 in]
            n148 = Index Array(array=w380) -> (element #1=w367:string, element #2=w376:string, element #3=w375:string)  [unwired: 3 in]
            n149 = Replace Array Subset(array=w382, new element=w366, index=6) -> (w369:string[])
            n150 = Replace Array Subset(array=w369, new element=w367, index=5) -> (w368:string[])
            n151 = Replace Array Subset(array=w368, new element=w376, index=7) -> (w379:string[])
            n152 = Replace Array Subset(array=w379, new element=w375, index=8) -> (w374:string[])
            n153 = Insert Into Array(array=w373, index (row)=w372, new element=w374) -> (w371:string[][])  [unwired: 1 in]
          }
          frame "Moved Up" {
            n154 = Delete From Array(array=w389, index (row)=w388) -> (deleted portion=w386:string[], array with subset deleted=w391:string[][])  [unwired: 2 in]
            n155 = Replace Array Subset(array=w386, new element=w385, index=6) -> (w383:string[])
            n156 = Decrement(x=w388) -> (x-1=w390:i32)
            n157 = Insert Into Array(array=w391, index (row)=w390, new element=w383) -> (w387:string[][])  [unwired: 1 in]
          }
          frame "Moved Down" {
            n158 = Delete From Array(array=w398, index (row)=w397) -> (deleted portion=w395:string[], array with subset deleted=w400:string[][])  [unwired: 2 in]
            n159 = Replace Array Subset(array=w395, new element=w394, index=6) -> (w392:string[])
            n160 = Increment(x=w397) -> (x+1=w399:i32)
            n161 = Insert Into Array(array=w400, index (row)=w399, new element=w392) -> (w396:string[][])  [unwired: 1 in]
          }
          frame "Deleted" {
            n162 = Delete From Array(array=w408, index (row)=w407) -> (deleted portion=w405:string[], array with subset deleted=w403:string[][])  [unwired: 2 in]
            n163 = Replace Array Subset(array=w405, new element=w404, index=6) -> (w402:string[])
            n164 = Build Array (concatenate)(w403, w402) -> (w401:string[][])
          }
          frame "Copied" {
            n165 = Delete From Array(array=w416, index (row)=w415) -> (deleted portion=w413:string[], array with subset deleted=w411:string[][])  [unwired: 2 in]
            n166 = Replace Array Subset(array=w413, new element=w412, index=6) -> (w410:string[])
            n167 = Build Array (concatenate)(w411, w410) -> (w409:string[][])
          }
        }
        n168 = Bundle By Name(cluster=w347, "New Step?"=FALSE, "Sequence History"=w343) -> (w349:T4)
      }
    }
  }
